vi "Program Gang.vi"(8 "error in (no error)":errorcluster, 9 "Micro":string, 10 "Active Positions":u32[](array[numeric]), 11 "Program Driver in":refnum<class "Program Driver.lvclass">) -> (0 "error out":errorcluster, 1 "Fail Codes":string[](array[string]), 2 "Tests Passed":bool[](array[boolean]), 3 "Program Driver out":refnum<class "Program Driver.lvclass">)   [LabVIEW 2015, in "Program Driver.lvclass"]
uses:
  Program Driver.lvclass
  Classes/Programmer/Programmer/Class/Programmer.lvclass
  <vilib>/Cree, Inc/Cree Test Framework/Classes/Base Objects/Base Class/Base Class/Base Class.lvclass
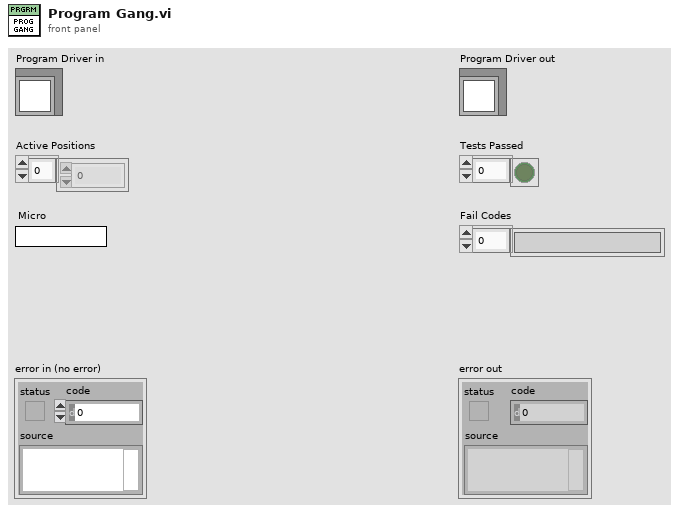
[diagram p1: front panel]
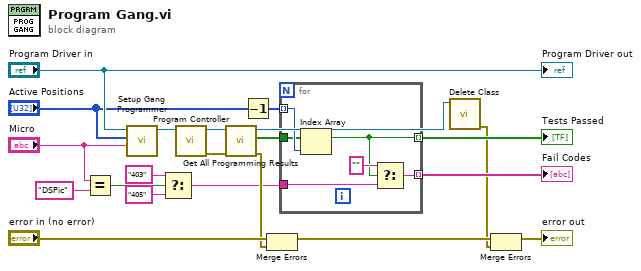
[diagram p0: block diagram]
diagram:
  n1 = Equal?(x="Micro", y="DSPic") -> (x = y?=w12:bool)
  n2 = call "Setup Gang Programmer.vi"("Chip"="Micro", "Active Positions"="Active Positions", "Test Template in"="Program Driver in") -> ("Programmer out"=w18:refnum<class "Programmer.lvclass">)  [unwired: 8 in]
  n3 = Select(t="403" ("y"), s=w12, f="405" ("y")) -> (s? t:f=w9:string)
  n4 = call-dynamic "Program Controller.vi"("Programmer in"=w18) -> ("error out"=w17:errorcluster, "Programmer out"=w19:refnum<class "Programmer.lvclass">)  [unwired: 9 in]
  n5 = call-dynamic "Get All Programming Results.vi"("error in (no error)"=w17, "Programmer in"=w19) -> ("error out"=w16:errorcluster, "Success"=w5:bool[], "Programmer out"=w4:refnum<class "Programmer.lvclass">)  [unwired: 6 in, 1 out]
  n6 = Decrement(x="Active Positions") -> (x-1=w6:u32[])
  n7 = Merge Errors("error in (no error)", w16) -> (w3:errorcluster)
  n8 = for {
    tunnel: w5 -> [w23]
    tunnel: [w22] -> w15 mode=indexing
    tunnel: w9 -> [w27]
    tunnel: [w25] -> w8 mode=indexing
    tunnel: w6 -> [w24] mode=indexing
    n9 = Index Array(array=w23, index=w24) -> (element=w22:bool)
    n10 = Select(t="", s=w22, f=w27) -> (s? t:f=w25:string)
  }
  "Tests Passed" <- w15
  "Fail Codes" <- w8
  n11 = call <vilib>:"Delete Class.vi"("Base Class in"=w4) -> ("error out"=w2:errorcluster)  [unwired: 9 in, 1 out]
  n12 = Merge Errors(w3, w2) -> (→"error out":errorcluster)
  "Program Driver out" <- "Program Driver in"
